vi "IO状态读取.vi"(8 "error in (no error)":errorcluster, 11 "Slave ID":T2) -> (0 "error out":errorcluster, 3 "STATES":T1)   [LabVIEW 2016, in "质控单元V1.lvlib"]
uses:
  <vilib>/Plasmionique/MB Master/MB_Master/MB_Master.lvclass
  <vilib>/Plasmionique/MB Master/MB Master.lvlib
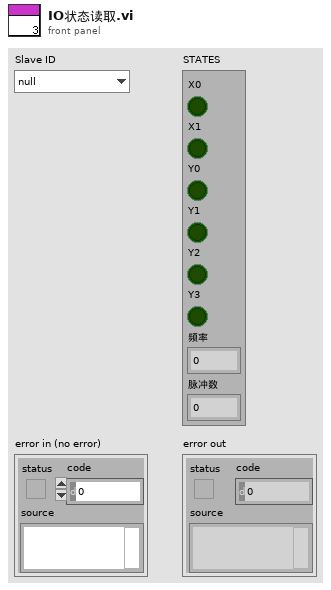
[diagram p1: front panel]
types:
  T1 = cluster{"X0":bool, "X1":bool, "Y0":bool, "Y1":bool, "Y2":bool, "Y3":bool, "频率":i32, "脉冲数":i32}
  T2 = typedef "质控单元V1.lvlib/质控slave id.ctl" = enum16{"null", "氨氮", "总磷", "CODMn", "CODCr", "总氮"}
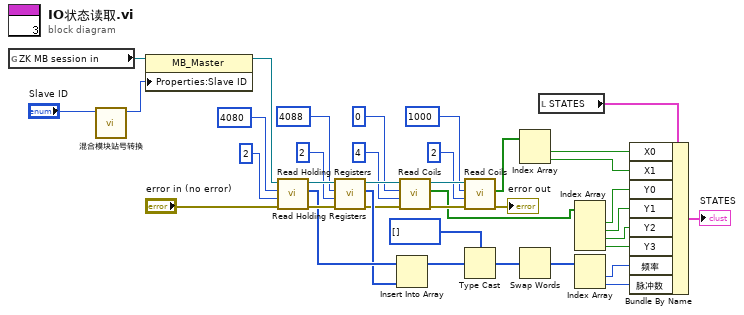
[diagram p0: block diagram]
diagram:
  n1 = global read "ZK非断电保存全局变量.vi" "ZK MB session in"() -> (w37:refnum<class "MB_Master.lvclass">)
  n2 = call "混合模块站号转换.vi"("Slave ID输入"="Slave ID") -> ("Slave ID输出"=w33:T2)  [unwired: 10 in]
  n3 = property class="MB_Master"(reference=w37, "Properties:Slave ID"=w33) -> (reference out=w36:refnum<class "MB_Master.lvclass">)  [unwired: 1 in, 1 out]
  n4 = call <vilib>:"Read Holding Registers.vi"("error in (no error)"="error in (no error)", "quantity"=u16 2, "starting address"=u16 4080, "MB session in"=w36) -> ("error out"=w31:errorcluster, "Registers"=w27:u16[], "MB session out"=w30:refnum<class "MB_Master.lvclass">)  [unwired: 5 in]
  n5 = call <vilib>:"Read Holding Registers.vi"("error in (no error)"=w31, "quantity"=u16 2, "starting address"=u16 4088, "MB session in"=w30) -> ("error out"=w21:errorcluster, "Registers"=w26:u16[], "MB session out"=w20:refnum<class "MB_Master.lvclass">)  [unwired: 5 in]
  n6 = Insert Into Array(array=w27, new element=w26) -> (w25:u16[])  [unwired: 1 in]
  n7 = call <vilib>:"Read Coils.vi"("error in (no error)"=w21, "quantity"=u16 4, "starting address"=u16 0, "MB session in"=w20) -> ("error out"=w15:errorcluster, "Coils"=w7:bool[], "MB session out"=w14:refnum<class "MB_Master.lvclass">)  [unwired: 5 in]
  n8 = call <vilib>:"Read Coils.vi"("error in (no error)"=w15, "quantity"=u16 2, "starting address"=u16 1000, "MB session in"=w14) -> ("error out"=→"error out":errorcluster, "Coils"=w10:bool[])  [unwired: 5 in, 1 out]
  n9 = Type Cast(type=i32[] [], x=w25) -> (*(type *) &x=w23:i32[])
  n10 = Index Array(array=w10) -> (element #1=w9:bool, element #2=w8:bool)  [unwired: 2 in]
  n11 = Swap Words(1:w23) -> (0:w22:i32[])
  n12 = local read "STATES"() -> (w17:T1)
  n13 = Index Array(array=w7) -> (element #1=w6:bool, element #2=w5:bool, element #3=w4:bool, element #4=w3:bool)  [unwired: 4 in]
  n14 = Index Array(array=w22) -> (element #1=w2:i32, element #2=w1:i32)  [unwired: 2 in]
  n15 = Bundle By Name(cluster=w17, "X0"=w9, "X1"=w8, "Y0"=w6, "Y1"=w5, "Y2"=w4, "Y3"=w3, "频率"=w2, "脉冲数"=w1) -> (→"STATES":T1)
